vi "Right Vector Check.vi"(8 "Column":i32, 9 "Row":i32, 10 "Opponent's Tiles":bool[][](array[boolean]), 11 "Current Player's Tiles":bool[][](array[boolean])) -> (2 "Possible Flips":T1[](array[typedef]), 3 "Possible Location":bool)   [LabVIEW 2020, in "Reversi.lvlib" / "Reversi.lvclass"]
uses:
  Reversi.lvclass
  Space Coordinates.ctl
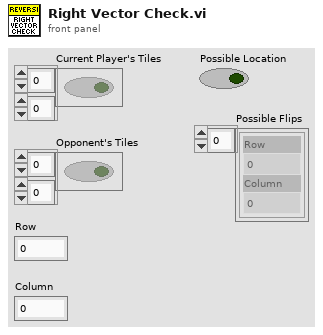
[diagram p1: front panel]
types:
  T1 = typedef "Reversi.lvlib/Reversi.lvclass/Space Coordinates.ctl" = cluster{"Row":i32, "Column":i32}
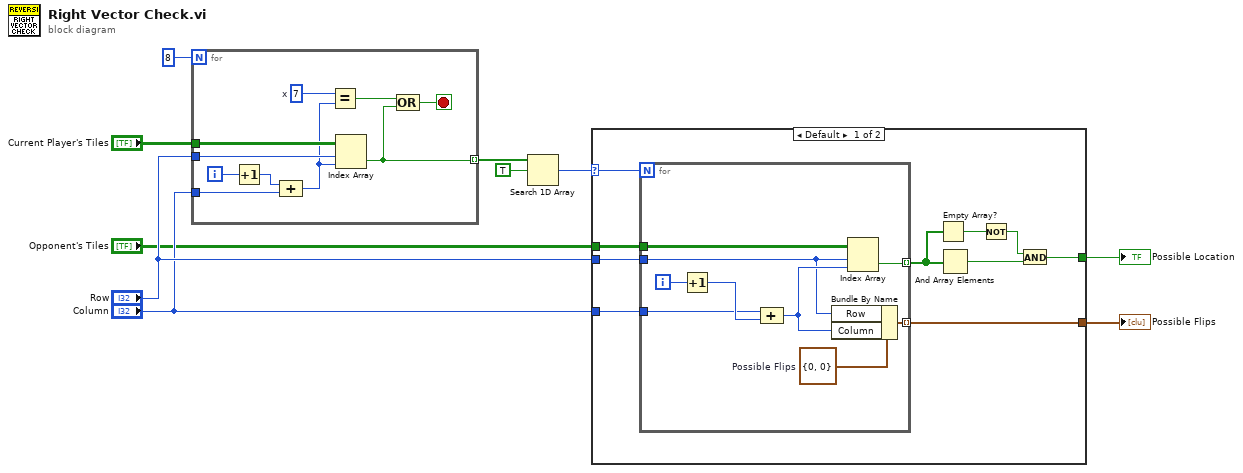
[diagram p0: block diagram]
diagram:
  n1 = for {
    N: 8 -> [_]
    tunnel: [w16] -> w9 mode=indexing
    tunnel: "Current Player's Tiles" -> [w20]
    tunnel: "Column" -> [w14]
    tunnel: "Row" -> [w13]
    i -> [w19]
    stop <- w15 stop-if-true
    w11 = 7  # x
    n2 = Increment(x=w19) -> (x+1=w18:i32)
    n3 = Compound Arithmetic op=ADD(w18, w14) -> (w12:i32)
    n4 = Equal?(x=w11, y=w12) -> (x = y?=w17:bool)
    n5 = Index Array(array=w20, index (row)=w13, index (col)=w12) -> (element=w16:bool)
    n6 = Compound Arithmetic op=OR(w17, w16) -> (w15:bool)
  }
  n7 = Search 1D Array(1D array=w9, element=TRUE) -> (index of element=w2:i32)  [unwired: 1 in]
  n8 = case shown="Default" w2 {
    selector: w2 -> [w21 _]
    tunnel: "Opponent's Tiles" -> [w26 _]
    tunnel: "Column" -> [w24 _]
    tunnel: [w27 _] -> w6
    tunnel: "Row" -> [w25 _]
    tunnel: [w22 _] -> w10
    frame Default {
      n9 = for {
        N: w21 -> [_]
        tunnel: [w37] -> w23 mode=indexing
        tunnel: w26 -> [w39]
        tunnel: w25 -> [w31]
        tunnel: w24 -> [w33]
        tunnel: [w35] -> w22 mode=indexing
        i -> [w38]
        w34 = T1 {"Row"=0, "Column"=0}  # Possible Flips
        n10 = Increment(x=w38) -> (x+1=w36:i32)
        n11 = Compound Arithmetic op=ADD(w33, w36) -> (w32:i32)
        n12 = Bundle By Name(cluster=w34, "Row"=w31, "Column"=w32) -> (w35:T1)
        n13 = Index Array(array=w39, index (row)=w31, index (col)=w32) -> (element=w37:bool)
      }
      n14 = Empty Array?(array=w23) -> (empty?=w30:bool)
      n15 = And Array Elements(Boolean array=w23) -> (logical AND=w28:bool)
      n16 = Not(x=w30) -> (.not. x?=w29:bool)
      n17 = And(x=w29, y=w28) -> (x .and. y?=w27:bool)
    }
    frame -1 {
    }
  }
  "Possible Flips" <- w10
  "Possible Location" <- w6
